vi "HornScan_Recipe_with_HornScan_SUB_VI.vi"(0 "connection ID":refnum<k5>, 2 "Receipe Msg ID":u32=31, 3 "Receipe Message length":u32=16, 4 "Response ID":i32=32, 5 "error in (no error)":errorcluster, 8 "Start Frequency":u32=19450, 9 "Time Delay":u16=70, 10 "Stop Frequency":u32=20449, 11 "Max Amplitude":u16=75, 12 "Frequency Step":u16=75, 13 "Max Current":u16=80) -> (14 "Pass":string="Horn Scan Success", 15 "connection ID_out":refnum<k5>, 16 "Resonant Frequencies":string, 19 "error out":errorcluster)   [LabVIEW 2017]
panel:
  in  "SetDigitalTuneWithHornScan":u16
  # "OUTPUT"
  # "INPUT"
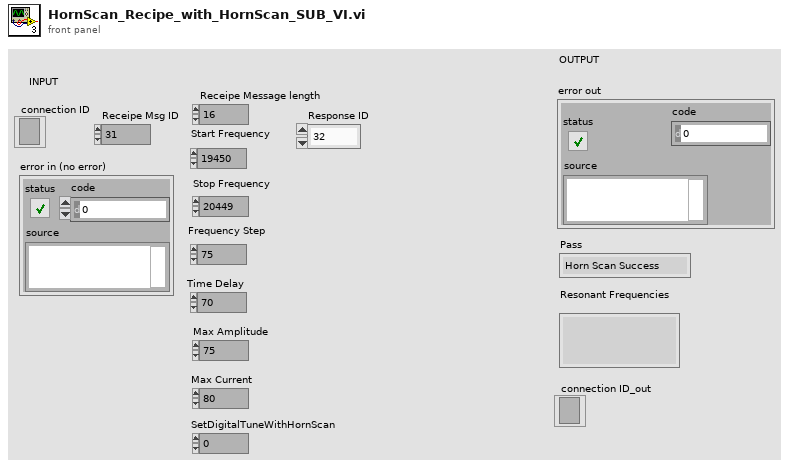
[diagram p1: front panel]
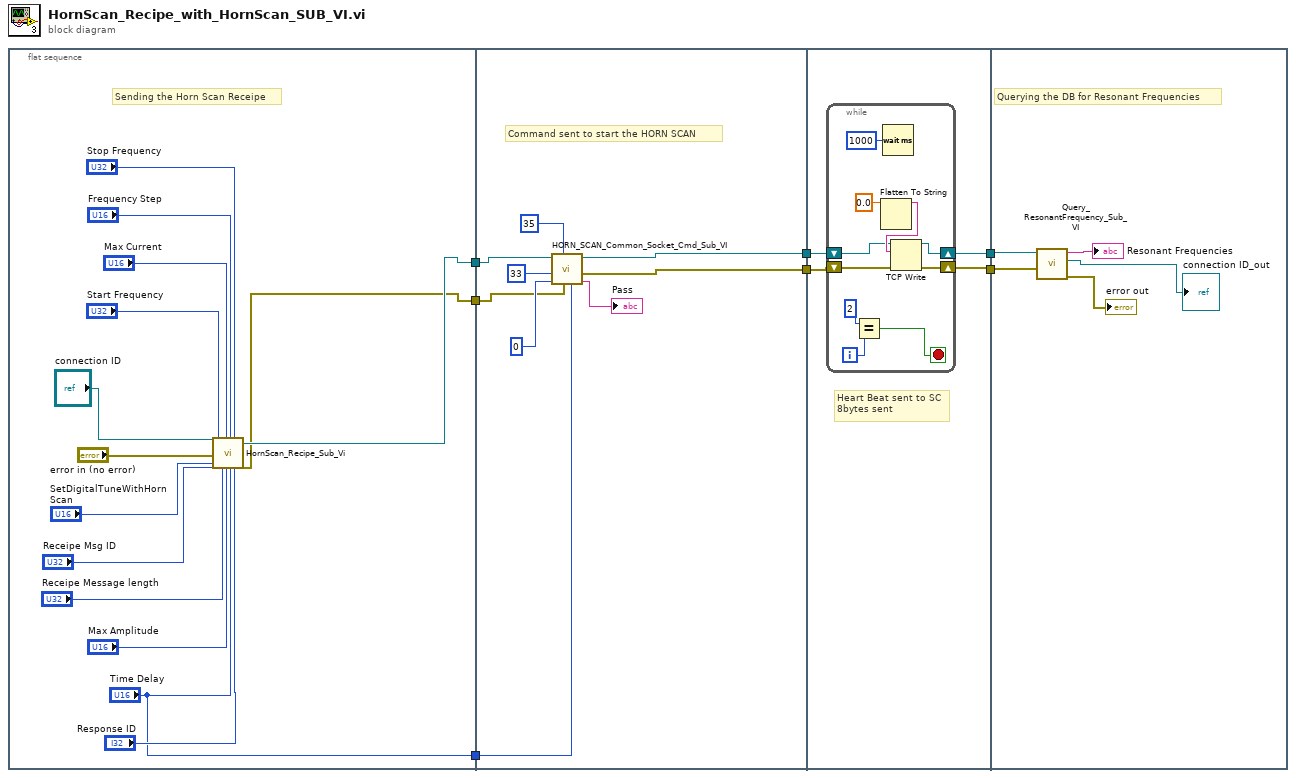
[diagram p0: block diagram]
diagram:
  n1 = flat-sequence {
    tunnel: ["Time Delay"] -> w3
    tunnel: [w9] -> w2
    tunnel: [w8] -> w1
    tunnel: [w26] -> w7
    tunnel: [w25] -> w5
    tunnel: w3 -> [w24]
    tunnel: w2 -> [w23]
    tunnel: w1 -> [w22]
    tunnel: w7 -> [w34]
    tunnel: [w33] -> w6
    tunnel: w5 -> [w32]
    tunnel: [w31] -> w4
    tunnel: w6 -> [w49]
    tunnel: w4 -> [w48]
    frame #0 {
      # "Sending the Horn Scan Receipe"
      n2 = call "HornScan_Recipe_Sub_Vi.vi"("connection ID"="connection ID", "error in (no error)"="error in (no error)", "SetDigitalTuneWithHornScan"="SetDigitalTuneWithHornScan", "Receipe Msg ID"="Receipe Msg ID", "Start Frequency"="Start Frequency", "Receipe Message length"="Receipe Message length", "Max Current"="Max Current", "Max Amplitude"="Max Amplitude", "Frequency Step"="Frequency Step", "Time Delay"="Time Delay", "Stop Frequency"="Stop Frequency", "Response ID"="Response ID") -> ("connection ID"=w9:refnum<k5>, "error out"=w8:errorcluster)  [unwired: 13 in, 1 out]
    }
    frame #1 {
      # "Command sent to start the HORN SCAN"
      n3 = call "HORN_SCAN_Common_Socket_Cmd_Sub_VI.vi"("Time Delay"=w24, "Common Socket Error in"=w22, "Response ID 1"=u8 35, "Operation Message Length"=0 ("Operation Message Length 1"), "Operation Message ID"=33 ("Operation Message ID 1"), "connection ID"=w23) -> ("Status"=→"Pass":string, "error out"=w25:errorcluster, "connection ID"=w26:refnum<k5>)  [unwired: 3 in]
    }
    frame #2 {
      # "Heart Beat sent to SC\n8bytes sent"
      n4 = while {
        shift-right: [w41] -> w33
        shift-left: w34 -> [w42]
        shift-right: [w39] -> w31
        shift-left: w32 -> [w40]
        i -> [w38]
        stop <- w35 stop-if-true
        n5 = Equal?(x=2, y=w38) -> (x = y?=w35:bool)
        n6 = Flatten To String(anything=0.0) -> (data string=w43:string)  [unwired: 3 in, 2 out]
        n7 = Wait (ms)(milliseconds to wait=u32 1000) -> ()  [unwired: 1 out]
        n8 = TCP Write(connection ID=w42, data in=w43, error in (no error)=w40) -> (connection ID out=w41:refnum<k5>, error out=w39:errorcluster)  [unwired: 1 in, 1 out]
      }
    }
    frame #3 {
      # "Querying the DB for Resonant Frequencies"
      n9 = call "Query_ResonantFrequency_Sub_VI.vi"("error in (no error)"=w48, "connection ID"=w49) -> ("error out"=→"error out":errorcluster, "connection ID_out"=→"connection ID_out":refnum<k5>, "Resonant Frequencies"=→"Resonant Frequencies":string)  [unwired: 7 in]
    }
  }
